vi "midtermV2.vi"() -> ()   [LabVIEW 2023]
panel:
  in  "Tab Control 2":enum32{"Data Collection", "Peak Finder"}(tab)
  in  "Time to Record (s)":dbl(slide)=1.0 scale=0.0..10.0
  in  "Capture Data":bool
  in  "Playback Peak\nFrequency":bool
  in  "Sampling \nFrequency (Hz)":dbl=44100.0
  out "Peak Frequency (Hz)":dbl
  in  "Device #":i32
  in  "#Peaks to\nLocate":i32=5
  in  "Exclusivity\nWidth (Hz)":dbl
  out "Peaks":dbl[](array[numeric])
  in  "Tab Control":enum32{"Raw Audio", "Power Spectrum"}(tab)
  out "Raw Audio":cluster{dbl[], "Array":dbl[]}(graph)
  out "Power Spectrum":waveform(dbl)(graph)
  in  "stop":bool
  # "Midterm Spectrum Analyzer"
  # "Ignore values\nwithin this range\nof a local maximum"
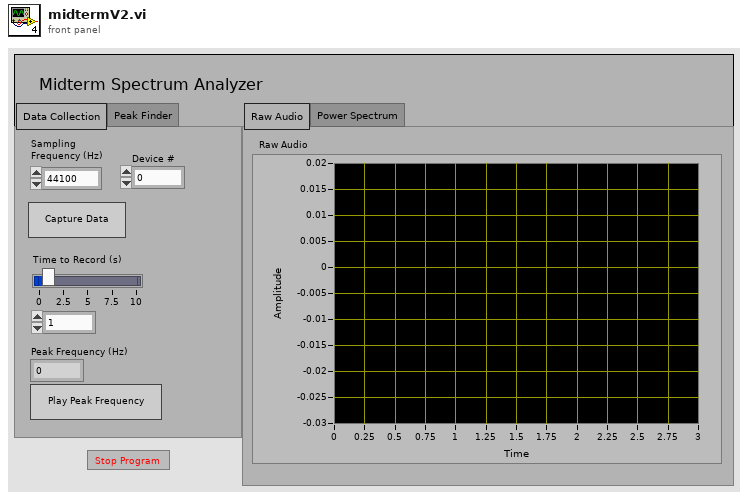
[diagram p1: front panel]
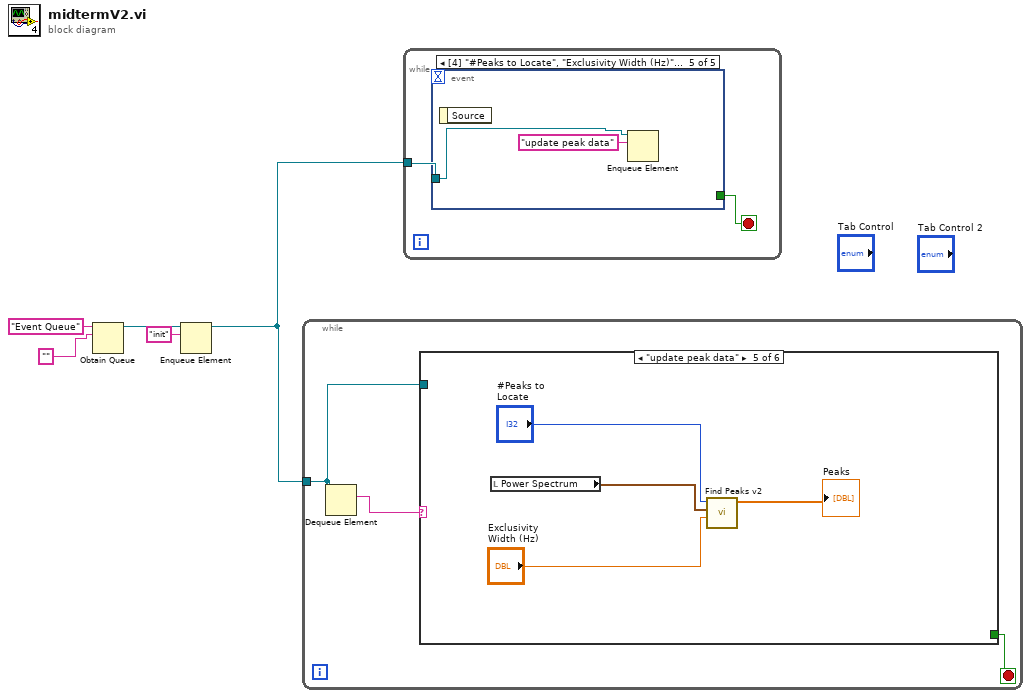
[diagram p0: block diagram]
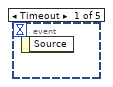
[diagram p2: hidden frame]
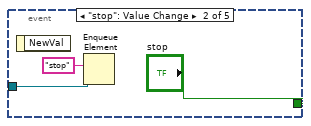
[diagram p3: hidden frame]
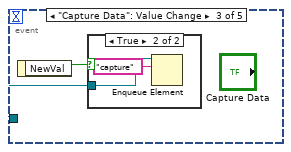
[diagram p4: hidden frame]
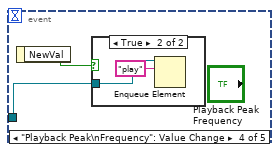
[diagram p6: hidden frame]
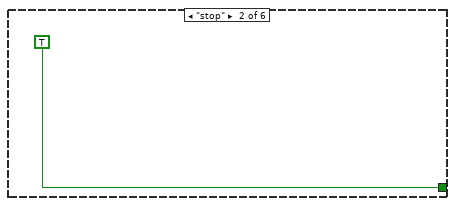
[diagram p9: hidden frame]
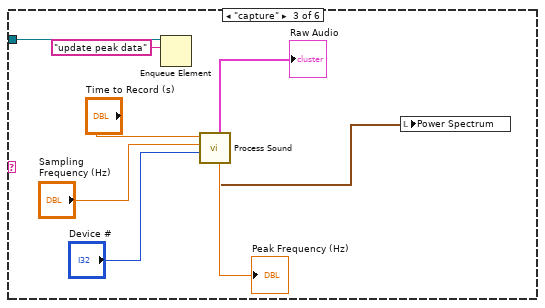
[diagram p10: hidden frame]
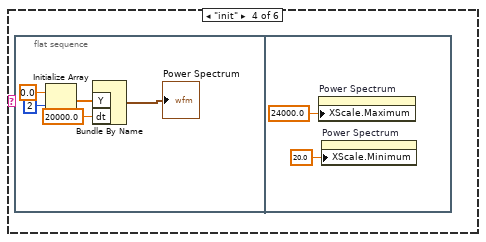
[diagram p11: hidden frame]
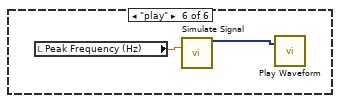
[diagram p12: hidden frame]
diagram:
  n1 = Obtain Queue(name (unnamed)="Event Queue", element data type="") -> (queue out=w3:refnum<queue>)  [unwired: 3 in, 2 out]
  n2 = Enqueue Element(queue=w3, element="init") -> (queue out=w2:refnum<queue>)  [unwired: 2 in, 2 out]
  n3 = while {
    tunnel: w2 -> [w6]
    stop <- w7 stop-if-true
    n4 = Dequeue Element(queue=w6) -> (element=w8:string)  [unwired: 2 in, 3 out]
    n5 = case shown="\"update peak data\"" w8 {
      tunnel: [_ TRUE _ _ _ _] -> w7
      tunnel: w6 -> [_ _ w17 _ _ _]
      frame "False", Default {
      }
      frame "stop" {
      }
      frame "capture" {
        n6 = Enqueue Element(queue=w17, element="update peak data") -> ()  [unwired: 2 in, 3 out]
        n7 = call "Process Sound.vi"("Device"="Device #", "Sampling \nFrequency (Hz)"="Sampling \nFrequency (Hz)", "Time to Record (s)"="Time to Record (s)") -> ("Peak Frequency"=→"Peak Frequency (Hz)":dbl, "Power Spectrum"=w10:waveform(dbl), "Sound Data"=→"Raw Audio":cluster{dbl[], "Array":dbl[]})  [unwired: 6 in]
        n8 = local write "Power Spectrum"(w10) -> ()
      }
      frame "init" {
        n9 = flat-sequence {
          frame #0 {
            n10 = Initialize Array(0.0 ("element"), 2 ("dimension size")) -> (w20:dbl[])
            n11 = Bundle By Name("Y"=w20, "dt"=20000.0) -> (→"Power Spectrum":waveform(dbl))  [unwired: 1 in]
          }
          frame #1 {
            n12 = property on="Power Spectrum" class="WFGraph (strict)"("XScale.Maximum"=24000.0 ("X Scale.Range:Maximum")) -> ()  [unwired: 2 in, 2 out]
            n13 = property on="Power Spectrum" class="WFGraph (strict)"("XScale.Minimum"=20.0 ("X Scale.Range:Minimum")) -> ()  [unwired: 2 in, 2 out]
          }
        }
      }
      frame "update peak data" {
        n14 = local read "Power Spectrum"() -> (w28:waveform(dbl))
        n15 = call "Find Peaks v2.vi"("Exclusivity Width (Hz)"="Exclusivity\nWidth (Hz)", "Power Spectrum"=w28, "#Peaks to Locate"="#Peaks to\nLocate") -> ("Array"=→"Peaks":dbl[])  [unwired: 8 in]
      }
      frame "play" {
        n16 = local read "Peak Frequency (Hz)"() -> (w30:dbl)
        n17 = call "Simulate Signal"("Frequency"=w30) -> ("Sine"=w29:dynamicdata)  [unwired: 13 in, 1 out]
        n18 = call "Play Waveform"("Data"=w29) -> ()  [unwired: 18 in, 1 out]
      }
    }
  }
  n19 = while {
    tunnel: w2 -> [w31]
    stop <- w32 stop-if-true
    n20 = event shown="[4] \"#Peaks to Locate\", \"Exclusivity Width (Hz)\": Value Change" {
      selector: _ -> [_ _ _ _ _]
      dyn-events: _ -> [_ _ _ _ _]
      timeout: _ -> [_ _ _ _ _]
      tunnel: [_ "stop" _ _ _] -> w32
      tunnel: w31 -> [_ w34 w36 w40 w44]
      event Timeout {
        n21 = event-data() -> ()  [unwired: 1 in, 1 out]
      }
      event "stop": Value Change {
        n22 = event-data() -> ()  [unwired: 1 in, 1 out]
        n23 = Enqueue Element(queue=w34, element="stop") -> ()  [unwired: 2 in, 3 out]
      }
      event "Capture Data": Value Change {
        n24 = event-data() -> ("NewVal"=w37:bool)  [unwired: 1 in]
        n25 = case shown="True" w37 {
          tunnel: w36 -> [_ w39]
          frame False {
          }
          frame True {
            n26 = Enqueue Element(queue=w39, element="capture") -> ()  [unwired: 2 in, 3 out]
          }
        }
      }
      event "Playback Peak\nFrequency": Value Change {
        n27 = event-data() -> ("NewVal"=w41:bool)  [unwired: 1 in]
        n28 = case shown="True" w41 {
          tunnel: w40 -> [_ w43]
          frame False {
          }
          frame True {
            n29 = Enqueue Element(queue=w43, element="play") -> ()  [unwired: 2 in, 3 out]
          }
        }
      }
      event "#Peaks to\nLocate", "Exclusivity\nWidth (Hz)": Value Change {
        n30 = event-data() -> ()  [unwired: 1 in, 1 out]
        n31 = Enqueue Element(queue=w44, element="update peak data") -> ()  [unwired: 2 in, 3 out]
      }
    }
  }
